vi "Element Type.vi"(11 "ButtonControl in":refnum<class "DigitalButtonControl.lvclass">) -> (2 "Element Type":string)   [LabVIEW 2020, in "VolatusGUIElements.lvlib" / "DigitalButtonControl.lvclass"]
uses:
  DigitalButtonControl.lvclass
  DigitalButtonControl.lvclass/DigitalButtonControl.ctl
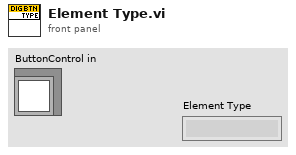
[diagram p1: front panel]
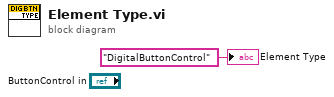
[diagram p0: block diagram]
diagram:
  "Element Type" <- "DigitalButtonControl" ("Element Type")
